vi "Shuffle one pair.vi"(10 "Array in":cluster{"String":string, "String 2":string}[](array[cluster]), 11 "Input":string) -> (3 "Array out":string[](array[string]))   [LabVIEW 2020]
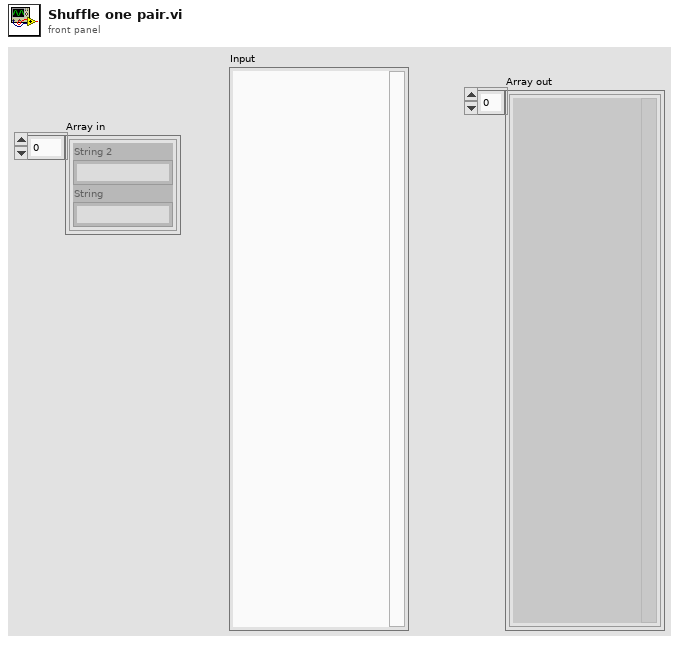
[diagram p1: front panel]
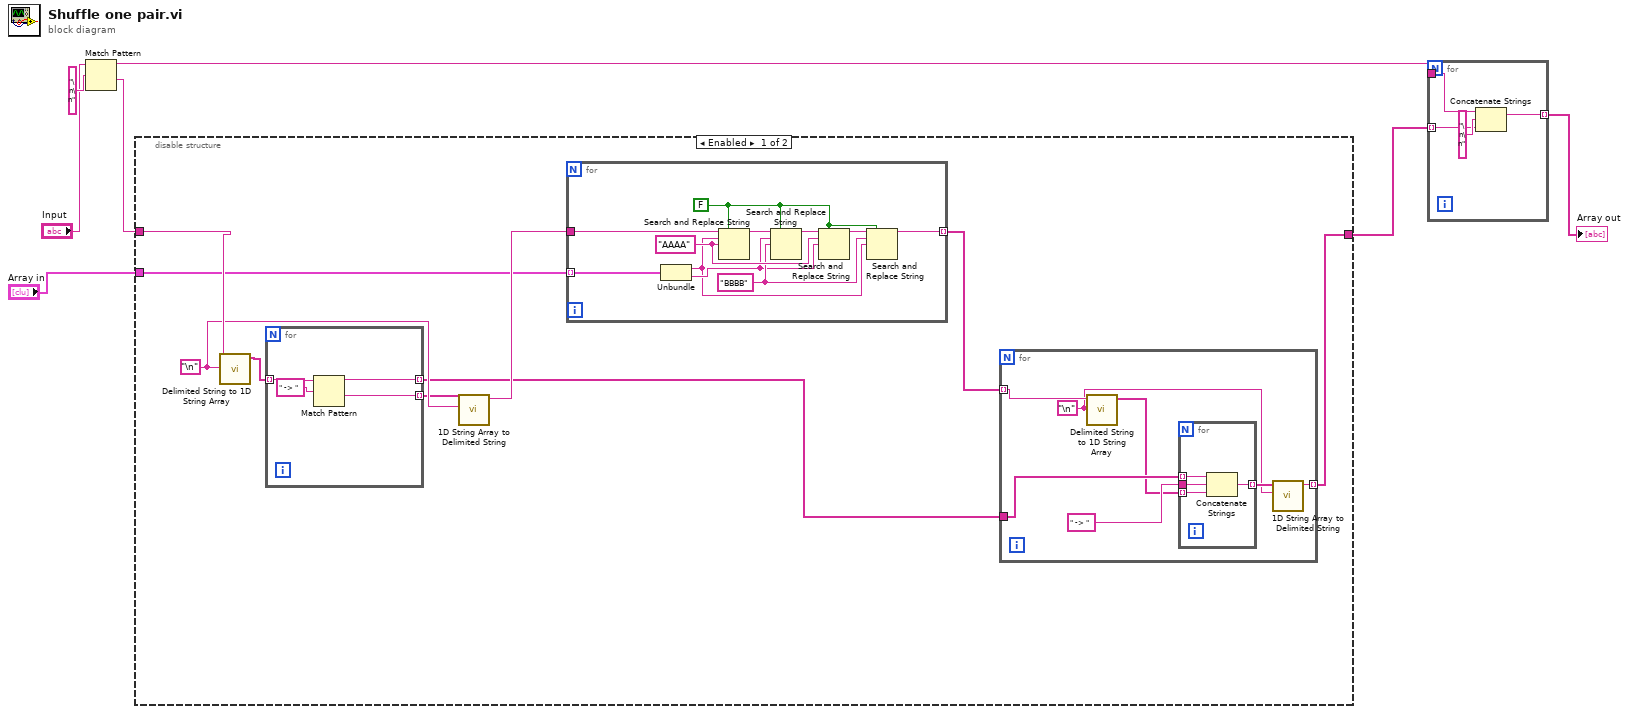
[diagram p0: block diagram]
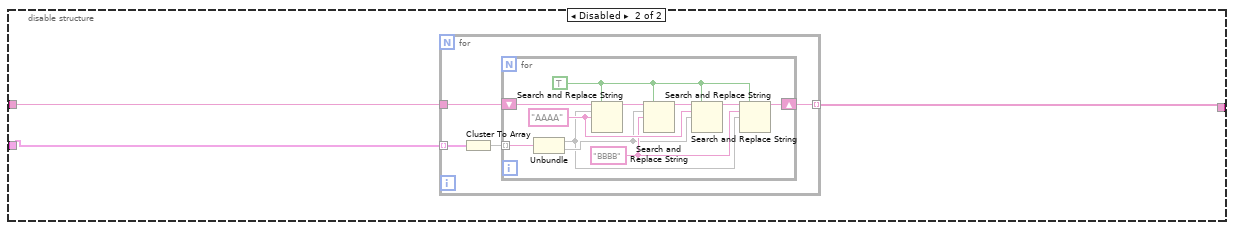
[diagram p2: hidden frame]
diagram:
  n1 = Match Pattern(string="Input", regular expression="\n\n") -> (before substring=w3:string, after substring=w4:string)  [unwired: 1 in, 2 out]
  n2 = disable-structure shown="Enabled" {
    disable-tunnel: w4 -> [w16 w44]
    disable-tunnel: [w10 w45] -> w2
    disable-tunnel: "Array in" -> [w9 w43]
    frame Enabled {
      w14 = "\n"
      n3 = call <vilib>:"Delimited String to 1D String Array.vi"("delimiter"=w14, "delimited string"=w16) -> ("string array"=w15:string[])  [unwired: 9 in]
      n4 = for {
        tunnel: w15 -> [w31] mode=indexing
        tunnel: [w29] -> w12 mode=indexing
        tunnel: [w28] -> w8 mode=indexing
        n5 = Match Pattern(string=w31, regular expression=" -> " ("delimiter")) -> (before substring=w29:string, after substring=w28:string)  [unwired: 1 in, 2 out]
      }
      n6 = call <vilib>:"1D String Array to Delimited String.vi"("delimiter"=w14, "string array"=w8) -> ("delimited string"=w13:string)  [unwired: 9 in]
      n7 = for {
        tunnel: w9 -> [w40] mode=indexing
        tunnel: w13 -> [w42]
        tunnel: [w41] -> w11 mode=indexing
        w32 = FALSE ("replace all? (F)")
        w38 = "BBBB" ("String")
        w39 = "AAAA"
        n8 = Unbundle(w40) -> ("String"=w36:string, "String 2"=w37:string)
        n9 = Search and Replace String(replace all?=w32, input string=w42, search string=w36, replace string=w39) -> (result string=w35:string)  [unwired: 4 in, 3 out]
        n10 = Search and Replace String(replace all?=w32, input string=w35, search string=w37, replace string=w38) -> (result string=w34:string)  [unwired: 4 in, 3 out]
        n11 = Search and Replace String(replace all?=w32, input string=w34, search string=w39, replace string=w37) -> (result string=w33:string)  [unwired: 4 in, 3 out]
        n12 = Search and Replace String(replace all?=w32, input string=w33, search string=w38, replace string=w36) -> (result string=w41:string)  [unwired: 4 in, 3 out]
      }
      n13 = for {
        tunnel: w11 -> [w23] mode=indexing
        tunnel: w12 -> [w22]
        tunnel: [w17] -> w10 mode=indexing
        w18 = "\n"
        n14 = call <vilib>:"Delimited String to 1D String Array.vi"("delimiter"=w18, "delimited string"=w23) -> ("string array"=w20:string[])  [unwired: 9 in]
        n15 = for {
          tunnel: w22 -> [w27] mode=indexing
          tunnel: " -> " ("delimiter") -> [w26]
          tunnel: w20 -> [w25] mode=indexing
          tunnel: [w24] -> w19 mode=indexing
          n16 = Concatenate Strings(w27, w26, w25) -> (w24:string)
        }
        n17 = call <vilib>:"1D String Array to Delimited String.vi"("delimiter"=w18, "string array"=w19) -> ("delimited string"=w17:string)  [unwired: 9 in]
      }
    }
    frame Disabled {
      n18 = for {
        tunnel: w43 -> [w49] mode=indexing
        tunnel: w44 -> [w48]
        tunnel: [w47] -> w45 mode=indexing
        n19 = Cluster To Array(cluster=w49) -> (array=w46:string[])
        n20 = for {
          tunnel: w46 -> [w57] mode=indexing
          shift-right: [w59] -> w47
          shift-left: w48 -> [w60]
          w55 = "BBBB" ("String")
          w56 = "AAAA"
          w58 = TRUE ("replace all? (F)")
          n21 = Unbundle(w57) -> (w53, w54)
          n22 = Search and Replace String(replace all?=w58, input string=w60, search string=w53, replace string=w56) -> (result string=w52:string)  [unwired: 4 in, 3 out]
          n23 = Search and Replace String(replace all?=w58, input string=w52, search string=w54, replace string=w55) -> (result string=w51:string)  [unwired: 4 in, 3 out]
          n24 = Search and Replace String(replace all?=w58, input string=w51, search string=w56, replace string=w54) -> (result string=w50:string)  [unwired: 4 in, 3 out]
          n25 = Search and Replace String(replace all?=w58, input string=w50, search string=w55, replace string=w53) -> (result string=w59:string)  [unwired: 4 in, 3 out]
        }
      }
    }
  }
  n26 = for {
    tunnel: w3 -> [w64]
    tunnel: w2 -> [w62] mode=indexing
    tunnel: [w61] -> w1 mode=indexing
    n27 = Concatenate Strings(w64, "\n\n" ("string"), w62) -> (w61:string)
  }
  "Array out" <- w1
